vi "Excel_Set_Chart_Colors.vi"(0 "Excel._Worksheet":refnum<k7>, 1 "MarkerStyle":i32(ring)=-4142 items=["xlMarkerStyleAutomatic"=-4105, "xlMarkerStyleCircle"=8, "xlMarkerStyleDash"=-4115, "xlMarkerStyleDiamond"=2, "xlMarkerStyleDot"=-4118, "xlMarkerStyleNone"=-4142, "xlMarkerStylePicture"=-4147, "xlMarkerStylePlus"=9, "xlMarkerStyleSquare"=1, "xlMarkerStyleStar"=5, "xlMarkerStyleTriangle"=3, "xlMarkerStyleX"=-4168], 2 "weight":i16=1, 5 "Shapes":refnum<k7>, 9 "chart index":i16=-1, 11 "error in (no error)":errorcluster, 12 "plot colors":u32[](array[colorbox]), 13 "plot area color":u32(colorbox)=16777215, 14 "chart area color":u32(colorbox)) -> (15 "error out":errorcluster)   [LabVIEW 2017, in "NI_ReportGenerationToolkit.lvlib"]
uses:
  <vilib>/addons/_office/NI_ReportGenerationToolkit.lvlib
panel:
  in  "Graph.Point":refnum<k7>
  in  "Excel._OLEObject":refnum<k7>
  in  "Graph.Chart":refnum<k7>
  in  "Graph.Series":refnum<k7>
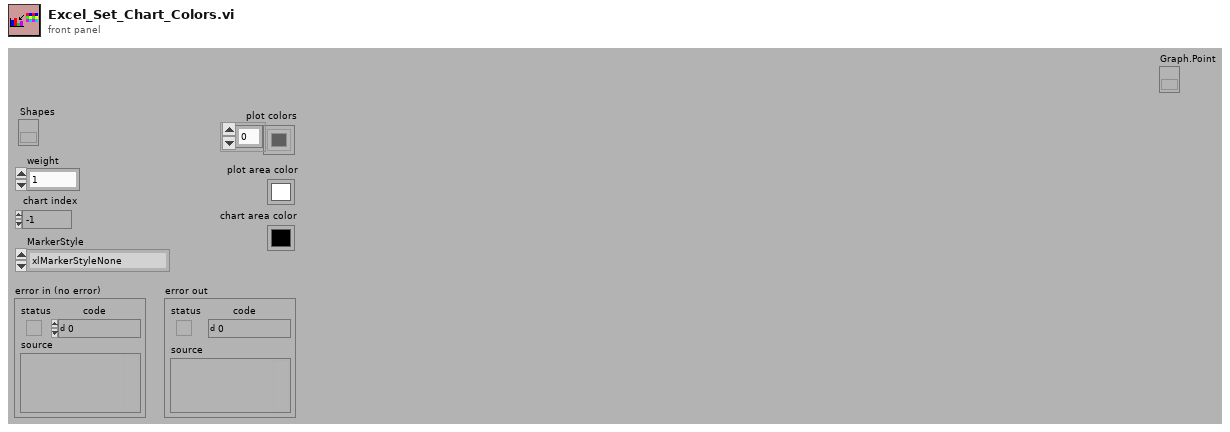
[diagram p1: front panel]
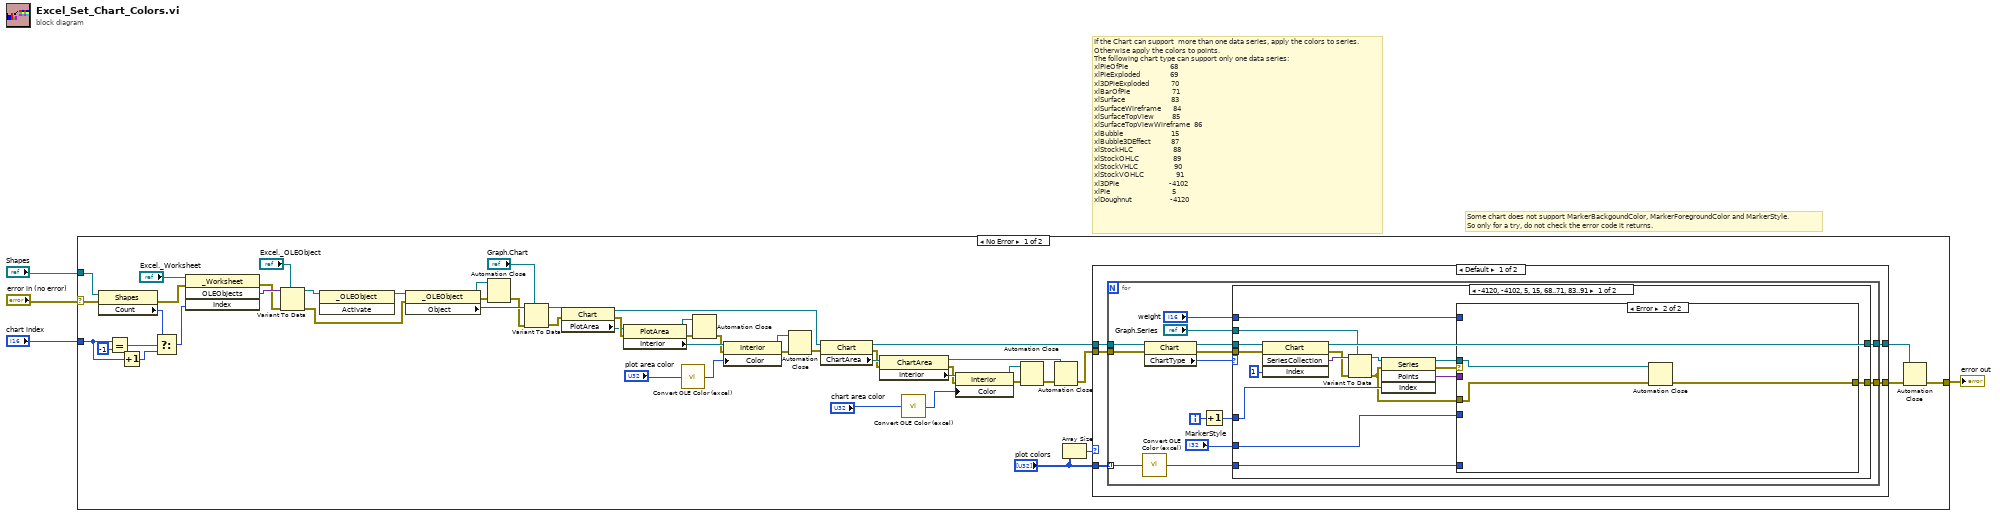
[diagram p0: block diagram]
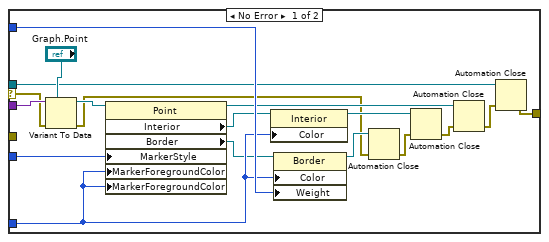
[diagram p2: hidden frame]
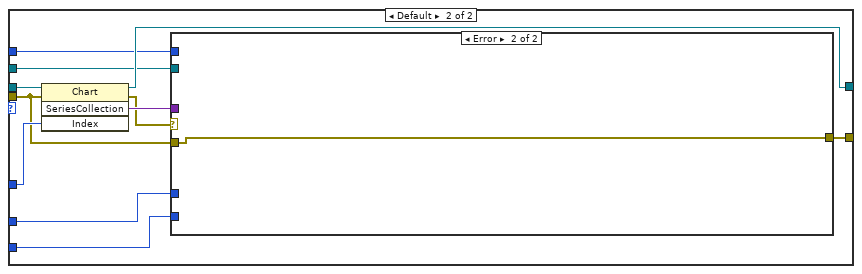
[diagram p3: hidden frame]
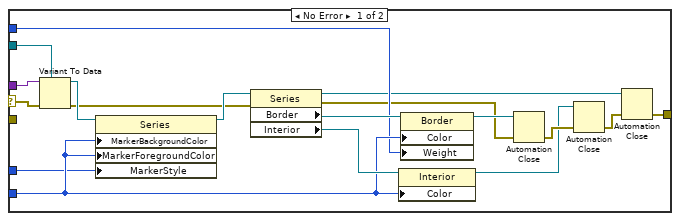
[diagram p4: hidden frame]
diagram:
  # "Some chart does not support MarkerBackgoundColor, MarkerForegroundColor and MarkerStyle. \nSo only for a try, do not check the error code it returns."
  # "If the Chart can support  more than one data series, apply the colors to series.\nOtherwise apply the colors to points.\nThe following chart type can support only one data series:\nxlPieOfPie                     68\nxlPieExploded               69\nxl3DPieExploded           70\nxlBarOfPie                     71\nxlSurface                       83\nxlSurfaceWireframe      84\nxlSurfaceTopView         85\nxlSurfaceTopViewWireframe  86\nxlBubble                        15\nxlBubble3DEffect          87\nxlStockHLC                    88\nxlStockOHLC                 89\nxlStockVHLC                  90\nxlStockVOHLC                91\nxl3DPie                         -4102\nxlPie                               5\nxlDoughnut                   -4120"
  n1 = case shown="No Error" "error in (no error)" {
    selector: "error in (no error)" -> [w5 w146]
    tunnel: "chart index" -> [w19 _]
    tunnel: [w9 w146] -> w3
    tunnel: "Shapes" -> [w7 _]
    frame No Error {
      n2 = property class="Shapes"(reference=w7, error in=w5) -> (error out=w18:errorcluster, "Count"=w17:i32)  [unwired: 1 out]
      n3 = Equal?(x=w19, y=i16 -1) -> (x = y?=w53:bool)
      n4 = Increment(x=w19) -> (x+1=w51:i16)
      n5 = Select(t=w17, s=w53, f=w51) -> (s? t:f=w16:i32)
      n6 = invoke class="_Worksheet" method="OLEObjects"(reference="Excel._Worksheet", error in=w18, "Index"=w16) -> (error out=w25:errorcluster, "OLEObjects"=w26:variant)  [unwired: 1 in, 2 out]
      n7 = Variant To Data(error in=w25, type="Excel._OLEObject", Variant=w26) -> (data=w13:refnum<k7>, error out=w12:errorcluster)
      n8 = invoke class="_OLEObject" method="Activate"(reference=w13) -> (reference out=w15:refnum<k7>)  [unwired: 2 in, 2 out]
      n9 = property class="_OLEObject"(reference=w15, error in=w12) -> (reference out=w20:refnum<k7>, error out=w22:errorcluster, "Object"=w27:variant)
      n10 = Automation Close(3:w22, 5:w20) -> (0:w21:errorcluster)
      n11 = Variant To Data(error in=w21, type="Graph.Chart", Variant=w27) -> (data=w24:refnum<k7>, error out=w23:errorcluster)
      n12 = property class="Chart"(reference=w24, error in=w23) -> (reference out=w39:refnum<k7>, error out=w55:errorcluster, "PlotArea"=w43:refnum<k7>)
      n13 = property class="PlotArea"(reference=w43, error in=w55) -> (reference out=w49:refnum<k7>, error out=w50:errorcluster, "Interior"=w48:refnum<k7>)
      n14 = call <vilib>:"Convert OLE Color (excel).vi"("color in"="plot area color") -> ("color out"=w54:u32)
      n15 = Automation Close(3:w50, 5:w49) -> (0:w47:errorcluster)
      n16 = property class="Interior"(reference=w48, error in=w47, "Color"=w54) -> (reference out=w45:refnum<k7>, error out=w46:errorcluster)
      n17 = Automation Close(3:w46, 5:w45) -> (0:w38:errorcluster)
      n18 = property class="Chart"(reference=w39, error in=w38) -> (reference out=w40:refnum<k7>, error out=w33:errorcluster, "ChartArea"=w42:refnum<k7>)
      n19 = property class="ChartArea"(reference=w42, error in=w33) -> (reference out=w30:refnum<k7>, error out=w32:errorcluster, "Interior"=w41:refnum<k7>)
      n20 = call <vilib>:"Convert OLE Color (excel).vi"("color in"="chart area color") -> ("color out"=w37:u32)
      n21 = property class="Interior"(reference=w41, error in=w32, "Color"=w37) -> (reference out=w31:refnum<k7>, error out=w34:errorcluster)
      n22 = Automation Close(3:w34, 5:w31) -> (0:w35:errorcluster)
      n23 = Automation Close(3:w35, 5:w30) -> (0:w29:errorcluster)
      n24 = Array Size(array="plot colors") -> (size(s)=w6:i32)
      n25 = case shown="Default" w6 {
        tunnel: "plot colors" -> [w61 _]
        tunnel: [w60 w144] -> w11
        tunnel: [w59 w145] -> w10
        tunnel: w40 -> [w58 w145]
        tunnel: w29 -> [w57 w144]
        frame Default {
          n26 = for {
            tunnel: w58 -> [w66]
            tunnel: w57 -> [w65]
            tunnel: [w71] -> w59
            tunnel: [w72] -> w60
            tunnel: w61 -> [w73] mode=indexing
            i -> [w75]
            n27 = call <vilib>:"Convert OLE Color (excel).vi"("color in"=w73) -> ("color out"=w70:u32)
            n28 = property class="Chart"(reference=w66, error in=w65) -> (reference out=w64:refnum<k7>, error out=w63:errorcluster, "ChartType"=w62:i32)
            n29 = Increment(x=w75) -> (x+1=w74:i32)
            n30 = case shown="-4120, -4102, 5, 15, 68..71, 83..91" w62 {
              tunnel: w63 -> [w88 w114]
              tunnel: w74 -> [w86 w123]
              tunnel: [w81 w122] -> w72
              tunnel: w64 -> [w89 w121]
              tunnel: [w85 w120] -> w71
              tunnel: w70 -> [w79 w119]
              tunnel: "Graph.Series" -> [w83 w118]
              tunnel: "weight" -> [w82 w117]
              tunnel: "MarkerStyle" -> [w78 w116]
              frame -4120, -4102, 5, 15, 68..71, 83..91 {
                n31 = invoke class="Chart" method="SeriesCollection"(reference=w89, error in=w88, "Index"=1) -> (reference out=w85:refnum<k7>, error out=w91:errorcluster, "SeriesCollection"=w92:variant)  [unwired: 1 in, 1 out]
                n32 = Variant To Data(error in=w91, type=w83, Variant=w92) -> (data=w87:refnum<k7>, error out=w76:errorcluster)
                n33 = invoke class="Series" method="Points"(reference=w87, error in=w76, "Index"=w86) -> (reference out=w80:refnum<k7>, error out=w77:errorcluster, "Points"=w84:variant)  [unwired: 1 in, 1 out]
                n34 = case shown="Error" w77 {
                  selector: w77 -> [w93 _]
                  tunnel: w84 -> [w110 _]
                  tunnel: w82 -> [w107 _]
                  tunnel: [w102 w112] -> w81
                  tunnel: w80 -> [w101 w113]
                  tunnel: w79 -> [w99 _]
                  tunnel: w78 -> [w96 _]
                  tunnel: w76 -> [_ w111]
                  frame No Error {
                    n35 = Variant To Data(error in=w93, type="Graph.Point", Variant=w110) -> (data=w100:refnum<k7>, error out=w94:errorcluster)
                    n36 = property class="Point"(reference=w100, "MarkerStyle"=w96, "MarkerForegroundColor"=w99, "MarkerForegroundColor"=w99) -> (reference out=w95:refnum<k7>, "Interior"=w97:refnum<k7>, "Border"=w98:refnum<k7>)  [unwired: 1 in, 1 out]
                    n37 = property class="Interior"(reference=w97, "Color"=w99) -> (reference out=w108:refnum<k7>)  [unwired: 1 in, 1 out]
                    n38 = property class="Border"(reference=w98, "Color"=w99, "Weight"=w107) -> (reference out=w106:refnum<k7>)  [unwired: 1 in, 1 out]
                    n39 = Automation Close(3:w94, 5:w106) -> (0:w104:errorcluster)
                    n40 = Automation Close(3:w104, 5:w108) -> (0:w105:errorcluster)
                    n41 = Automation Close(3:w105, 5:w95) -> (0:w103:errorcluster)
                    n42 = Automation Close(3:w103, 5:w101) -> (0:w102:errorcluster)
                  }
                  frame Error {
                    n43 = Automation Close(3:w111, 5:w113) -> (0:w112:errorcluster)
                  }
                }
              }
              frame Default {
                n44 = invoke class="Chart" method="SeriesCollection"(reference=w121, error in=w114, "Index"=w123) -> (reference out=w120:refnum<k7>, error out=w115:errorcluster, "SeriesCollection"=w124:variant)  [unwired: 1 in, 1 out]
                n45 = case shown="Error" w115 {
                  selector: w115 -> [w125 _]
                  tunnel: w124 -> [w142 _]
                  tunnel: [w136 w143] -> w122
                  tunnel: w119 -> [w135 _]
                  tunnel: w118 -> [w133 _]
                  tunnel: w117 -> [w132 _]
                  tunnel: w116 -> [w131 _]
                  tunnel: w114 -> [_ w143]
                  frame No Error {
                    n46 = Variant To Data(error in=w125, type=w133, Variant=w142) -> (data=w139:refnum<k7>, error out=w130:errorcluster)
                    n47 = property class="Series"(reference=w139, "MarkerBackgroundColor"=w135, "MarkerForegroundColor"=w135, "MarkerStyle"=w131) -> (reference out=w138:refnum<k7>)  [unwired: 1 in, 1 out]
                    n48 = property class="Series"(reference=w138, error in=w130) -> (reference out=w127:refnum<k7>, error out=w128:errorcluster, "Border"=w134:refnum<k7>, "Interior"=w137:refnum<k7>)
                    n49 = property class="Interior"(reference=w137, "Color"=w135) -> (reference out=w126:refnum<k7>)  [unwired: 1 in, 1 out]
                    n50 = property class="Border"(reference=w134, "Color"=w135, "Weight"=w132) -> (reference out=w140:refnum<k7>)  [unwired: 1 in, 1 out]
                    n51 = Automation Close(3:w128, 5:w140) -> (0:w141:errorcluster)
                    n52 = Automation Close(3:w141, 5:w126) -> (0:w129:errorcluster)
                    n53 = Automation Close(3:w129, 5:w127) -> (0:w136:errorcluster)
                  }
                  frame Error {
                  }
                }
              }
            }
          }
        }
        frame 0 {
        }
      }
      n54 = Automation Close(3:w11, 5:w10) -> (0:w9:errorcluster)
    }
    frame Error {
    }
  }
  "error out" <- w3
